vi "AuMT8852B Inquiry Results Query.vi"(8 "error in (no error)":errorcluster, 11 "VISA session":refnum<visa-resource-name>) -> (0 "error out":errorcluster, 2 "error code":i32, 3 "VISA session out":refnum<visa-resource-name>, 4 "Addresses":string[](array[string]), 6 "Names":string[](array[string]))   [LabVIEW 2017]
doc: "Anritsu MT8852B Bluetooth Tester\n\nReturns the results of the address inquiry.\n\nOUTPUTS\nAddresses - list of all Bluetooth devices found.\nNames - user-friendly name (20 characters max) for each Bluetooth device found."
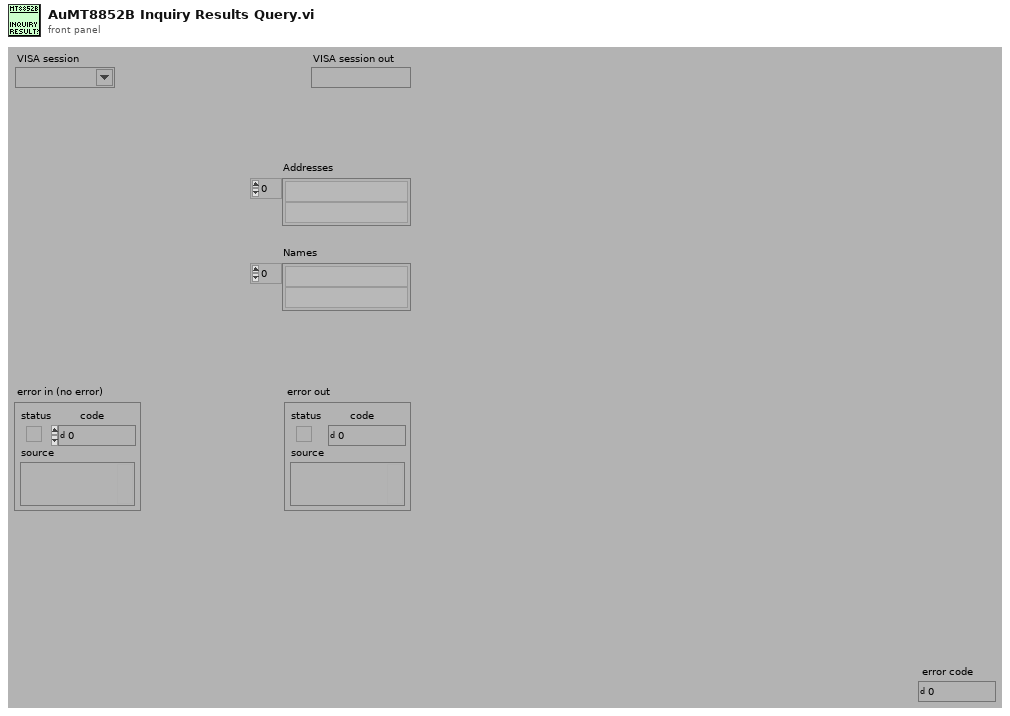
[diagram p1: front panel]
types:
  T1 = enum16{"Simulate", "Range check", "Cache", "Query instrument status"}
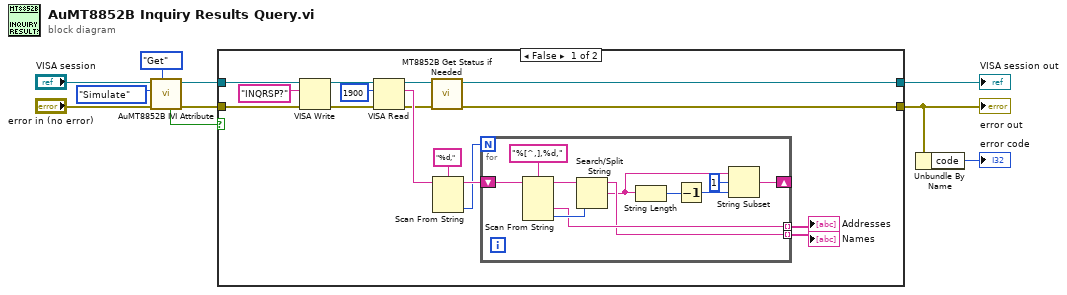
[diagram p0: block diagram]
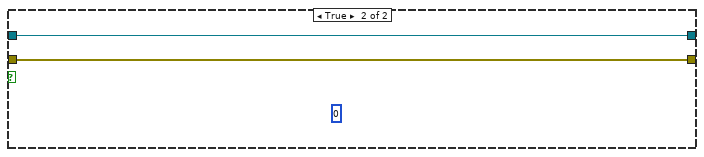
[diagram p2: hidden frame]
diagram:
  n1 = call <instrlib>:"AuMT8852B IVI Attribute.vi"("Set/Get (Set)"=enum16{"Set", "Get"}."Get", "error in (no error)"="error in (no error)", "Flag (Simulate)"=T1."Simulate", "VISA session"="VISA session") -> ("error out"=w7:errorcluster, "VISA session out"=w9:refnum<visa-resource-name>, "Value out"=w3:bool)  [unwired: 5 in]
  n2 = case shown="False" w3 {
    tunnel: [w20 w39] -> w10
    tunnel: [w19 w38] -> w1
    tunnel: w9 -> [w25 w39]
    tunnel: w7 -> [w24 w38]
    frame False {
      n3 = VISA Write(VISA resource name=w25, write buffer="INQRSP?" ("write buffer (\"\")"), error in (no error)=w24) -> (VISA resource name out=w23:refnum<visa-resource-name>, error out=w22:errorcluster)  [unwired: 1 out]
      n4 = VISA Read(VISA resource name=w23, byte count=u32 1900 ("byte count (0)"), error in (no error)=w22) -> (VISA resource name out=w18:refnum<visa-resource-name>, read buffer=w14:string, error out=w13:errorcluster)  [unwired: 1 out]
      n5 = call <instrlib>:"MT8852B Get Status if Needed.vi"("error in (no error)"=w13, "VISA session"=w18) -> ("error out"=w19:errorcluster, "VISA session out"=w20:refnum<visa-resource-name>)  [unwired: 8 in]
      n6 = Scan From String(format string="%d,", input string=w14) -> (remaining string=w17:string, output 1=w16:i32)  [unwired: 3 in, 2 out]
      n7 = for {
        N: w16 -> [_]
        shift-right: [w31] -> _
        shift-left: w17 -> [w34]
        tunnel: [w33] -> w12 mode=indexing
        tunnel: [w32] -> w11 mode=indexing
        n8 = Scan From String(format string="%[^,],%d," ("Format String"), input string=w34) -> (remaining string=w36:string, output 1=w33:string, output 2=w35:i32)  [unwired: 4 in, 2 out]
        n9 = Search/Split String(string=w36, offset (0)=w35) -> (substring before match=w32:string, match + rest of string=w29:string)  [unwired: 1 in, 1 out]
        n10 = String Length(string=w29) -> (length=w30:i32)
        n11 = Decrement(x=w30) -> (x-1=w28:i32)
        n12 = String Subset(string=w29, offset (0)=1, length (rest)=w28) -> (substring=w31:string)
      }
      "Addresses" <- w12
      "Names" <- w11
    }
    frame True {
      (unwired) u8 0
    }
  }
  "error out" <- w1
  "VISA session out" <- w10
  n13 = Unbundle By Name(w1) -> ("code"=→"error code":i32)
